vi "Controller Constructor.vi"(9 "Model.lvclass":refnum<class "Model.lvclass">, 10 "View.lvclass":refnum<class "View.lvclass">) -> (3 "Controller Out":refnum<class "Controller.lvclass">)   [LabVIEW 2016, in "Controller.lvclass"]
uses:
  Controller.lvclass
  View/View.lvclass
  Model/Model.lvclass
  Controller.lvclass/Controller.ctl
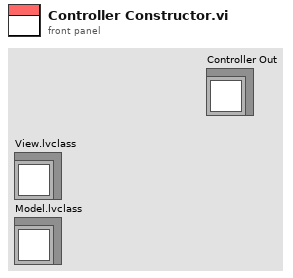
[diagram p1: front panel]
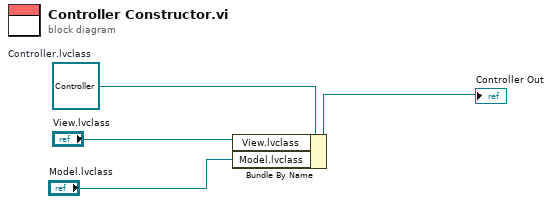
[diagram p0: block diagram]
diagram:
  w4 = refnum<class "Controller.lvclass"> refnum  # Controller.lvclass
  n1 = Bundle By Name(cluster=w4, "View.lvclass"="View.lvclass", "Model.lvclass"="Model.lvclass") -> (→"Controller Out":refnum<class "Controller.lvclass">)
